vi "CPP_SpeedRamp.vi"() -> (5 "Plug in titles":string[](array[string]), 7 "Plug in values":string[](array[string]))   [LabVIEW 2018]
panel:
  in  "Close This VI After Running?":bool=TRUE
  # "This VI now just calls \"SpeedRamp.vi\"."
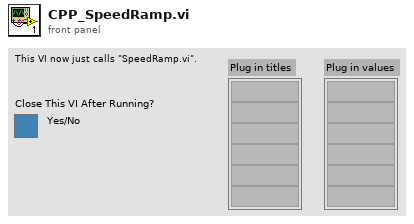
[diagram p1: front panel]
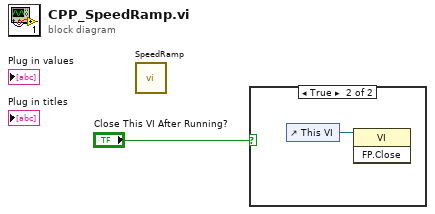
[diagram p0: block diagram]
diagram:
  n1 = call "SpeedRamp.vi"() -> ()  [unwired: 6 in, 2 out]
  n2 = case shown="True" "Close This VI After Running?" {
    frame False {
    }
    frame True {
      n3 = control-ref of="This VI"() -> (w2:refnum<vi>)
      n4 = invoke class="VI" method="FP.Close"(reference=w2) -> ()  [unwired: 2 in, 3 out]
    }
  }
